vi "myRIO__convert__FPGAvalue_to_Voltage__PortC.vi"(11 "input_FPGAvalue_PortC":i32) -> (3 "output_voltage":dbl)   [LabVIEW 2014]
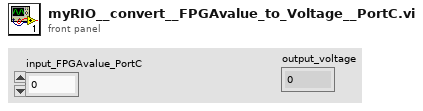
[diagram p1: front panel]
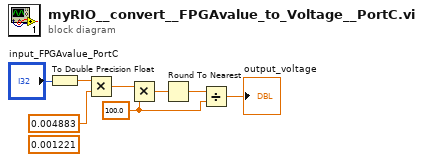
[diagram p0: block diagram]
diagram:
  w3 = 100.0 ("y")
  (unwired) 0.001221 ("f")
  n1 = To Double Precision Float(number="input_FPGAvalue_PortC") -> (double precision float=w7:dbl)
  n2 = Multiply(x=w7, y=0.004883 ("f")) -> (x*y=w6:dbl)
  n3 = Multiply(x=w6, y=w3) -> (x*y=w5:dbl)
  n4 = Round To Nearest(number=w5) -> (nearest integer value=w4:dbl)
  n5 = Divide(x=w4, y=w3) -> (x/y=→"output_voltage":dbl)
